vi "FTW-Actor-Log-Error.vi"(0 "FTW Actor Instance":refnum<class "FTW-ActorInstance.lvclass">, 5 "Explanation":string, 11 "Error to Log":errorcluster) -> (4 "FTW Actor Instance out":refnum<class "FTW-ActorInstance.lvclass">, 6 "Exception Occurred?":bool, 8 "Exception":T1, 10 "Serialized Event":string)   [LabVIEW 2012, in "FTW-Actor.lvlib" / "FTW-ActorInstance.lvclass"]
uses:
  FTW-ActorInstance.lvclass
  Core/src/Error/FTW-ERR-ExceptionType.ctl
panel:
  # "Inputs"
  # "Outputs"
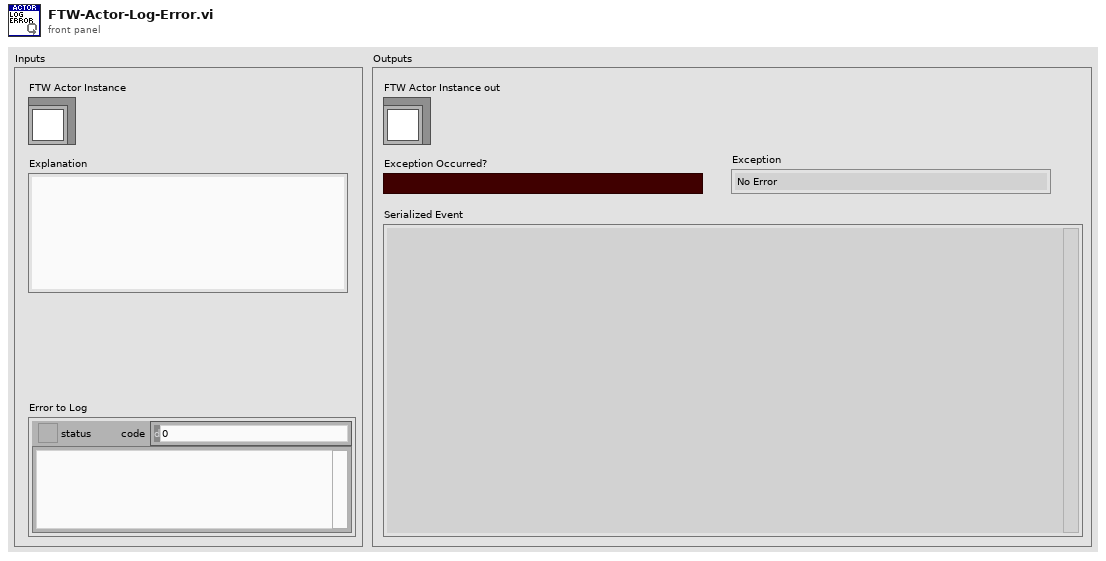
[diagram p1: front panel]
types:
  T1 = typedef "FTW-ERR-ExceptionType.ctl" = enum16{"No Error", "Error", "Warning"}
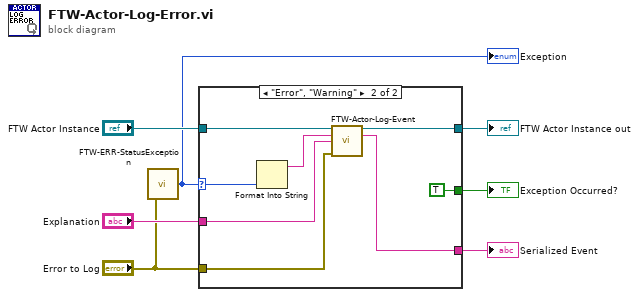
[diagram p0: block diagram]
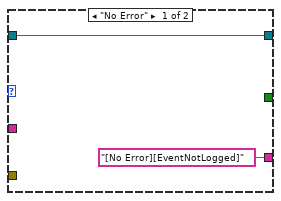
[diagram p2: hidden frame]
diagram:
  n1 = call "FTW-ERR-StatusException.vi"("error to check"="Error to Log") -> ("Exception"=w2:T1)
  "Exception" <- w2
  n2 = case shown="\"Error\", \"Warning\"" w2 {
    selector: w2 -> [_ w13]
    tunnel: "Error to Log" -> [_ w11]
    tunnel: "FTW Actor Instance" -> [w9 w16]
    tunnel: [w9 w15] -> w6
    tunnel: [_ TRUE] -> w5
    tunnel: "Explanation" -> [_ w12]
    tunnel: ["[No Error][EventNotLogged]" ("Serialized Event") w10] -> w1
    frame "No Error" {
    }
    frame "Error", "Warning" {
      n3 = Format Into String(w13) -> (resulting string=w14:string)  [unwired: 3 in, 1 out]
      n4 = call-dynamic "FTW-Actor-Log-Event.vi"("FTW Actor Instance"=w16, "Event Type"=w14, "Event Data"=w12, "error in"=w11) -> ("FTW Actor Instance out"=w15:refnum<class "FTW-ActorInstance.lvclass">, "Serialized Event"=w10:string)  [unwired: 9 in, 1 out]
    }
  }
  "FTW Actor Instance out" <- w6
  "Exception Occurred?" <- w5
  "Serialized Event" <- w1
